vi "Get Channel Name.vi"(8 "error in (no error)":errorcluster, 10 "channel index (1)":i32=1 caption="Channel Index (1)", 11 "CS++DCPwr in":refnum<class "CS++DCPwr.lvclass">) -> (0 "error out":errorcluster, 2 "channel name":string caption="Channel Name", 3 "CS++DCPwr out":refnum<class "CS++DCPwr.lvclass">)   [LabVIEW 2015, in "CS++DCPwr.lvlib" / "CS++DCPwr.lvclass"]
doc: "This VI returns the highest-level channel name that corresponds to the specific driver channel string that is in the channel table at an index you specify."
uses:
  CS++DCPwr.lvclass
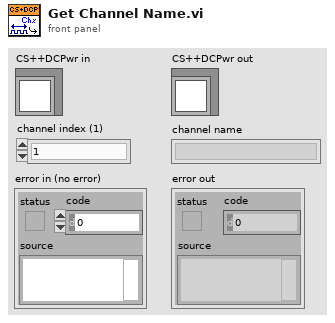
[diagram p1: front panel]
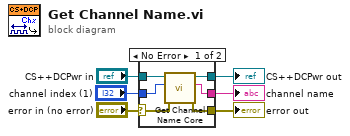
[diagram p0: block diagram]
diagram:
  n1 = case shown="No Error" "error in (no error)" {
    selector: "error in (no error)" -> [w9 w14]
    tunnel: [w8 w14] -> w5
    tunnel: [w11 w13] -> w3
    tunnel: "CS++DCPwr in" -> [w12 w13]
    tunnel: "channel index (1)" -> [w10 _]
    tunnel: [w7 _] -> w1
    frame No Error {
      n2 = call-dynamic "Get Channel Name Core.vi"("error in (no error)"=w9, "channel index (1)"=w10, "CS++DCPwr in"=w12) -> ("error out"=w8:errorcluster, "channel name"=w7:string, "CS++DCPwr out"=w11:refnum<class "CS++DCPwr.lvclass">)  [unwired: 6 in]
    }
    frame Error {
    }
  }
  "error out" <- w5
  "CS++DCPwr out" <- w3
  "channel name" <- w1
